vi "Read Include Result.vi"(8 "error in (no error)":errorcluster, 11 "JsonReportPlugin in":refnum<class "JsonReportPlugin.lvclass">) -> (0 "error out":errorcluster, 2 "Include Result":bool, 3 "JsonReportPlugin out":refnum<class "JsonReportPlugin.lvclass">)   [LabVIEW 2015, in "JsonReportPlugin.lvclass"]
uses:
  JsonReportPlugin.lvclass
  JsonReportPlugin.lvclass/JsonReportPlugin.ctl
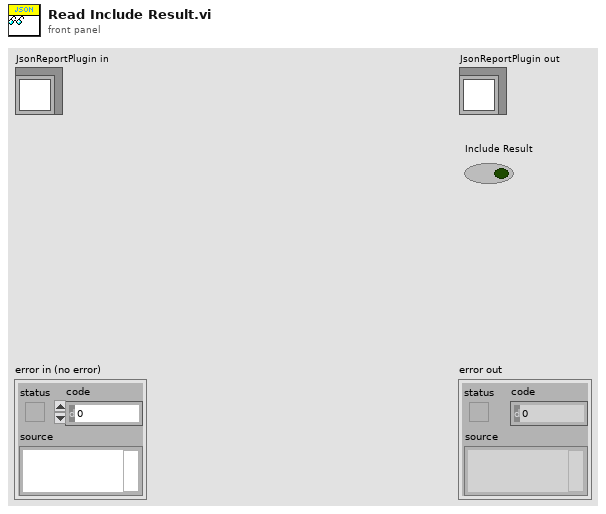
[diagram p1: front panel]
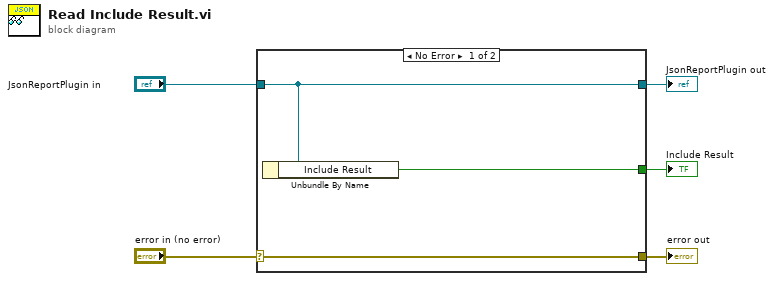
[diagram p0: block diagram]
diagram:
  n1 = case shown="No Error" "error in (no error)" {
    selector: "error in (no error)" -> [w8 w9]
    tunnel: [w8 w9] -> w4
    tunnel: [w7 w10] -> w2
    tunnel: "JsonReportPlugin in" -> [w7 w10]
    tunnel: [w6 _] -> w1
    frame No Error {
      n2 = Unbundle By Name(w7) -> ("Include Result"=w6:bool)
    }
    frame Error {
    }
  }
  "error out" <- w4
  "JsonReportPlugin out" <- w2
  "Include Result" <- w1
